vi "Data2Memory.vi"(0 "VNA Visa":refnum<visa-resource-name>, 11 "error in":errorcluster, 12 "Channel":i32, 13 "Radio Buttons":T1(radio)) -> (4 "VNA Visa Out":refnum<visa-resource-name>, 15 "error out":errorcluster)   [LabVIEW 2018, in "PNA-X.lvlib"]
uses:
  PNA-X.lvlib
panel:
  # "NORMal\n Trace data only\n \n ADD\n Data + Memory\n \n SUBTract\n Data - Memory\n \n MULTiply\n Data * Memory\n \n DIVide\n Data / Memory"
  # "Save  Data to Memory \nThen Exexute  Math"
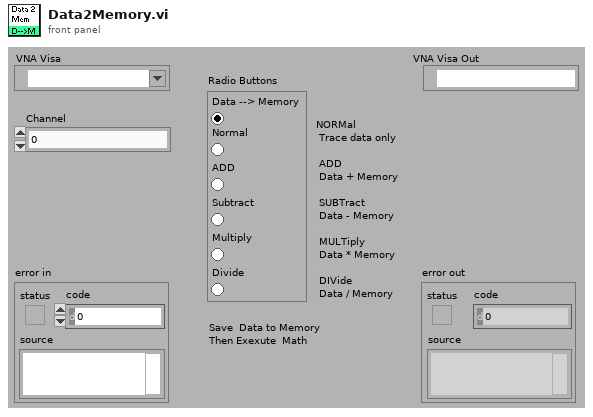
[diagram p1: front panel]
types:
  T1 = enum32{"Data --> Memory", "Normal", "ADD", "Subtract", "Multiply", "Divide"}
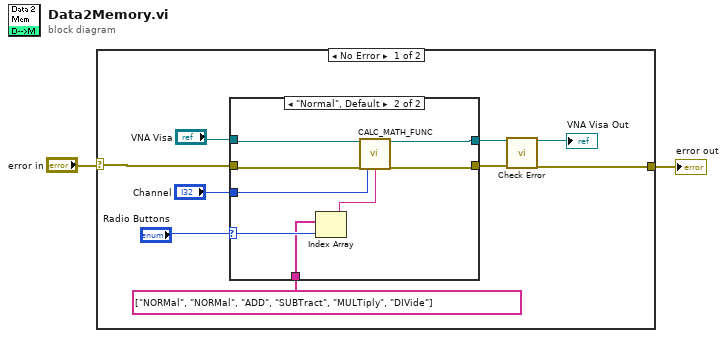
[diagram p0: block diagram]
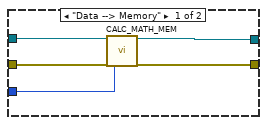
[diagram p2: hidden frame]
diagram:
  n1 = case shown="No Error" "error in" {
    selector: "error in" -> [w3 w25]
    tunnel: [w4 w25] -> w2
    frame No Error {
      n2 = case shown="\"Normal\", Default" "Radio Buttons" {
        selector: "Radio Buttons" -> [_ w21]
        tunnel: w3 -> [w16 w23]
        tunnel: "VNA Visa" -> [w15 w24]
        tunnel: "Channel" -> [w14 w22]
        tunnel: [w13 w19] -> w7
        tunnel: [w12 w18] -> w6
        tunnel: string[] ["NORMal", "NORMal", "ADD", "SUBTract", "MULTiply", "DIVide"] ("Functions") -> [_ w20]
        frame "Data --> Memory" {
          n3 = call "CALC_MATH_MEM.vi"("VISA IN"=w15, "error in"=w16, "Channel"=w14) -> ("VISA Out"=w12:refnum<visa-resource-name>, "error out"=w13:errorcluster)  [unwired: 15 in]
        }
        frame "Normal", Default {
          n4 = Index Array(array=w20, index=w21) -> (element=w17:string)
          n5 = call "CALC_MATH_FUNC.vi"("VISA IN"=w24, "error in"=w23, "Channel"=w22, "Combo Box"=w17) -> ("VISA Out"=w18:refnum<visa-resource-name>, "error out"=w19:errorcluster)  [unwired: 14 in]
        }
      }
      n6 = call "Check Error.vi"("VISA Resource Name"=w6, "error in (no error)"=w7) -> ("dup VISA session"=→"VNA Visa Out":refnum<visa-resource-name>, "error out"=w4:errorcluster)  [unwired: 16 in]
    }
    frame Error {
    }
  }
  "error out" <- w2
